vi "信道.vi"(2 "噪声标准差":dbl, 3 "调制信号":dbl[](array[numeric])) -> (0 "高斯噪声信号":dbl[](array[numeric]), 1 "信道输出信号":dbl[](array[numeric]))   [LabVIEW 2011]
uses:
  <vilib>/Analysis/NI_AALBase.lvlib
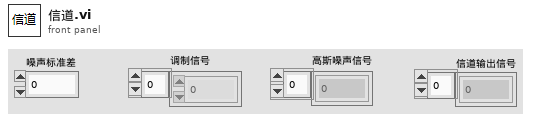
[diagram p1: front panel]
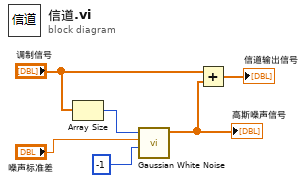
[diagram p0: block diagram]
diagram:
  n1 = Array Size(array="调制信号") -> (size(s)=w5:i32)
  n2 = call <vilib>:"Gaussian White Noise.vi"("seed"=-1, "standard deviation"="噪声标准差", "samples"=w5) -> ("Gaussian noise pattern"=w3:dbl[])  [unwired: 7 in, 1 out]
  "高斯噪声信号" <- w3
  n3 = Add(x="调制信号", y=w3) -> (x+y=→"信道输出信号":dbl[])
